vi "Test-XBoxController-Virtual.vi"() -> ()   [LabVIEW 2013]
uses:
  Robot/Virtual Systems/Tracer-V/Tracer-V.lvclass
  Robot/Logical Systems/TraceMessage/Trace.lvclass
  Robot/Virtual Systems/XBoxController-V/XboxController-V.lvclass
  <vilib>/ActorFramework/Message Queue/Message Queue.lvclass/Message Queue.ctl
  <vilib>/ActorFramework/Message Enqueuer/Message Enqueuer.lvclass/Message Enqueuer.ctl
  <vilib>/ActorFramework/Message Enqueuer/Enqueue.vi
  <vilib>/ActorFramework/Message Priority Queue/Priority Enqueue.vi
  Robot/Logical Systems/XBoxController Messages/Teleop Msg/Teleop Msg.lvclass
  <vilib>/ActorFramework/Stop Msg/Stop Msg.lvclass
  <vilib>/ActorFramework/Actor/Actor.lvclass
  <vilib>/ActorFramework/Message Queue/Message Queue.lvclass
panel:
  in  "stop 2":bool
  in  "DQ milliseconds to wait":u32=20
  out "# elements in queue":i32
  in  "Operator Controller":T1 {"Right Joystick Right" scale=-1.0..1.0; "Left Joystick Right" scale=-1.0..1.0; "Right Joystick Forward" scale=-1.0..1.0; "Left Joystick Forward" scale=-1.0..1.0}
  out "Log Time Stamp":timestamp
  out "Trace TimeTick":u32
  out "Message":string
  out "SourceVI":string
  in  "Driver Controller":T1 {"Right Joystick Right" scale=-1.0..1.0; "Left Joystick Right" scale=-1.0..1.0; "Right Joystick Forward" scale=-1.0..1.0; "Left Joystick Forward" scale=-1.0..1.0}
  in  "milliseconds to wait":u32=50
  in  "stop":bool
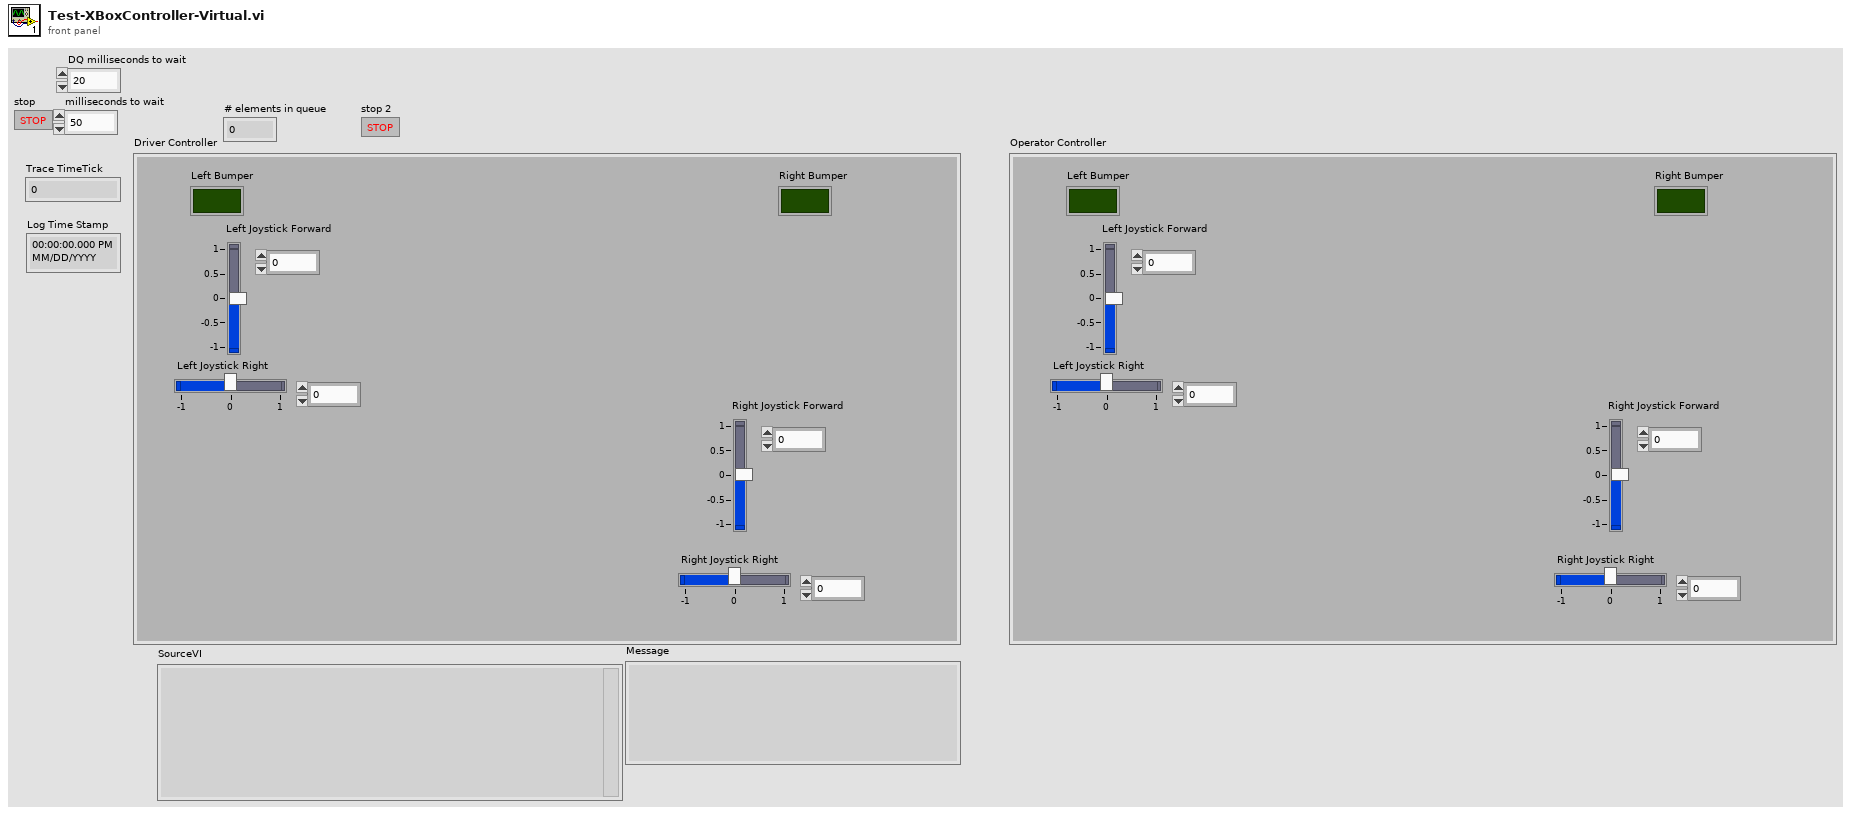
[diagram p1: front panel]
types:
  T1 = cluster{"Left Bumper":bool, "Right Bumper":bool, "Left Joystick Forward":dbl, "Left Joystick Right":dbl, "Right Joystick Forward":dbl, "Right Joystick Right":dbl}
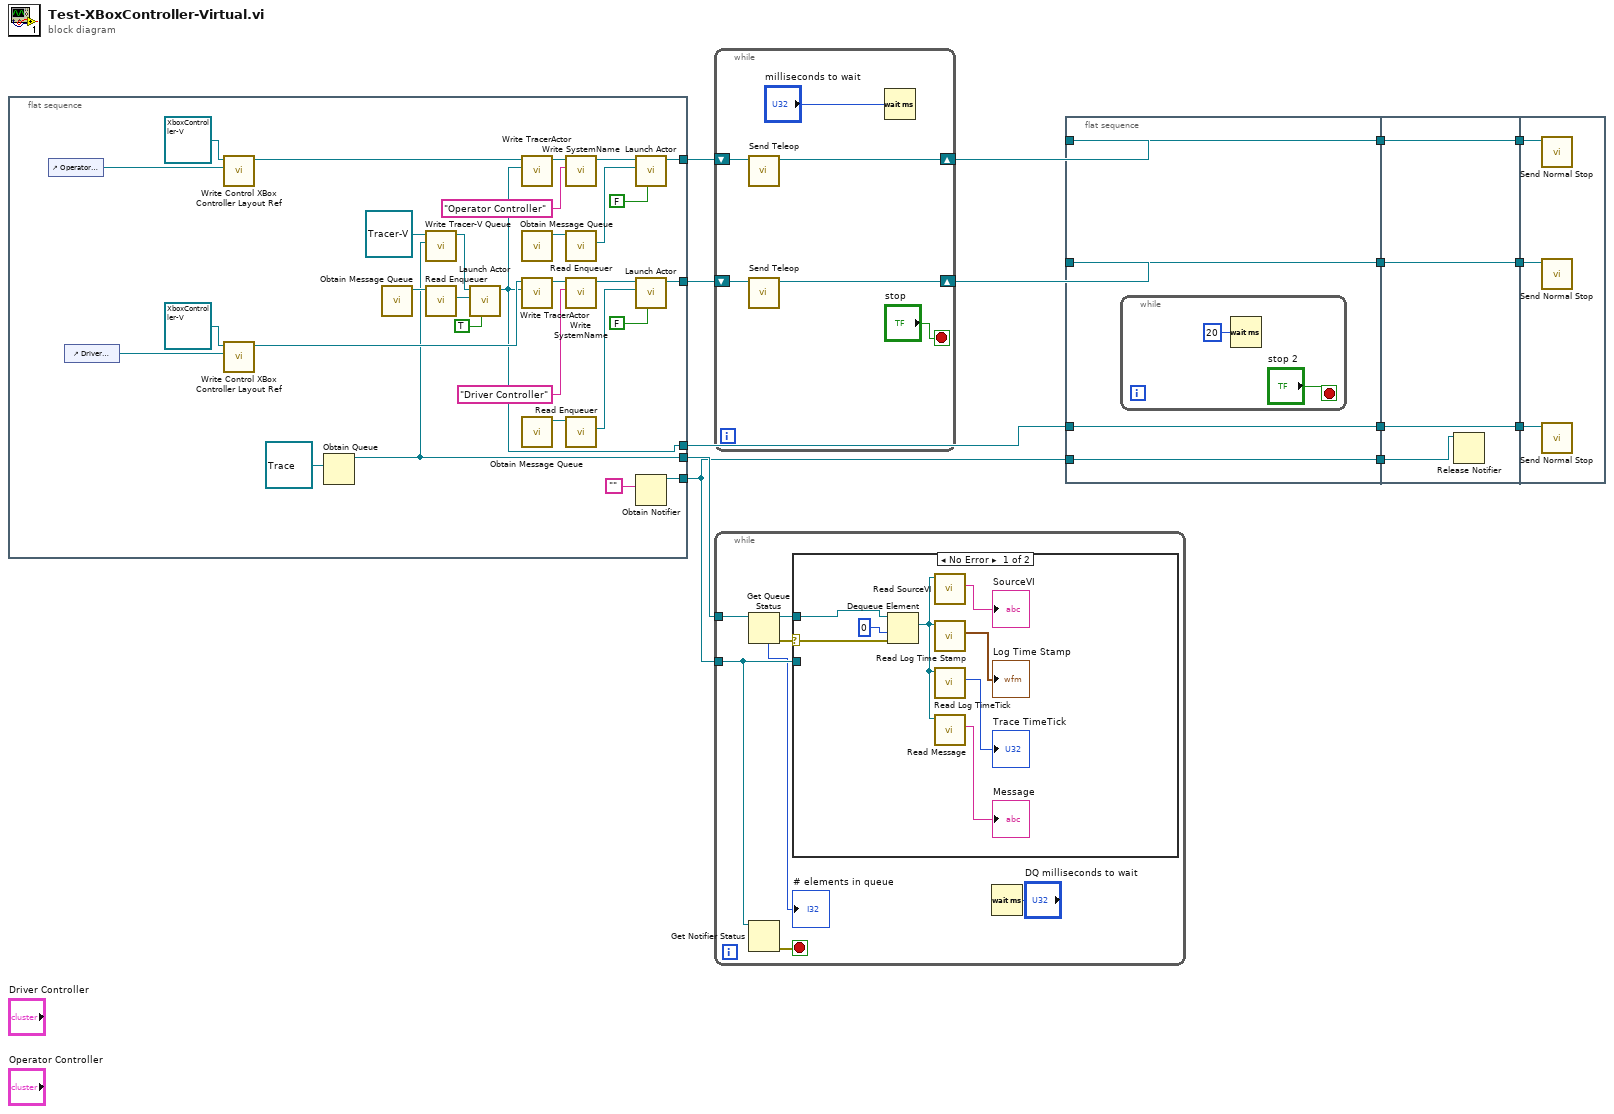
[diagram p0: block diagram]
diagram:
  n1 = flat-sequence {
    tunnel: [w42] -> w14
    tunnel: [w26] -> w12
    tunnel: [w29] -> w9
    tunnel: [w20] -> w11
    tunnel: [w17] -> w5
    frame #0 {
      n2 = control-ref of="Operator Controller"() -> (w27:refnum<vi>)
      n3 = control-ref of="Driver Controller"() -> (w39:refnum<vi>)
      n4 = call-dynamic "Write Control XBox Controller Layout Ref.vi"("XBox Controller Layout Ref"=w27, "XboxController-V in"=refnum<class "XboxController-V.lvclass"> refnum ("XboxController-V.lvclass")) -> ("XboxController-V out"=w25:refnum<class "XboxController-V.lvclass">)  [unwired: 8 in, 1 out]
      n5 = call-dynamic "Write Control XBox Controller Layout Ref.vi"("XBox Controller Layout Ref"=w39, "XboxController-V in"=refnum<class "XboxController-V.lvclass"> refnum ("XboxController-V.lvclass")) -> ("XboxController-V out"=w33:refnum<class "XboxController-V.lvclass">)  [unwired: 8 in, 1 out]
      n6 = Obtain Queue(element data type=refnum<class "Trace.lvclass"> refnum ("Trace.lvclass")) -> (queue out=w29:refnum<queue>)  [unwired: 4 in, 2 out]
      n7 = call <vilib>:"Obtain Message Queue.vi"() -> ("Message Queue"=w35:refnum<class "Message Queue.lvclass">)  [unwired: 10 in, 1 out]
      n8 = call-dynamic "Write Tracer-V Queue.vi"("TraceMessage Queue"=w29, "Tracer-V in"=refnum<class "Tracer-V.lvclass"> refnum ("Tracer-V.lvclass")) -> ("Tracer-V out"=w30:refnum<class "Tracer-V.lvclass">)  [unwired: 8 in, 1 out]
      n9 = call <vilib>:"Read Enqueuer.vi"("Message Queue"=w35) -> ("Message Enqueuer"=w34:refnum<class "Message Enqueuer.lvclass">)  [unwired: 10 in]
      n10 = call <vilib>:"Launch Actor.vi"("Open Actor Core front panel? (F)"=TRUE, "Actor-to-Caller Enqueuer"=w34, "Actor"=w30) -> ("Caller-To-Actor Enqueuer"=w26:refnum<class "Message Enqueuer.lvclass">)  [unwired: 7 in, 1 out]
      n11 = call-dynamic "Write TracerActor.vi"("Tracer"=w26, "System in"=w25) -> ("System out"=w24:refnum<class "XboxController-V.lvclass">)  [unwired: 8 in, 1 out]
      n12 = call <vilib>:"Obtain Message Queue.vi"() -> ("Message Queue"=w22:refnum<class "Message Queue.lvclass">)  [unwired: 10 in, 1 out]
      n13 = call-dynamic "Write TracerActor.vi"("Tracer"=w26, "System in"=w33) -> ("System out"=w36:refnum<class "XboxController-V.lvclass">)  [unwired: 8 in, 1 out]
      n14 = call <vilib>:"Obtain Message Queue.vi"() -> ("Message Queue"=w44:refnum<class "Message Queue.lvclass">)  [unwired: 10 in, 1 out]
      n15 = call-dynamic "Write SystemName.vi"("SystemName"="Operator Controller", "System in"=w24) -> ("System out"=w23:refnum<class "XboxController-V.lvclass">)  [unwired: 8 in, 1 out]
      n16 = call <vilib>:"Read Enqueuer.vi"("Message Queue"=w22) -> ("Message Enqueuer"=w21:refnum<class "Message Enqueuer.lvclass">)  [unwired: 10 in]
      n17 = call-dynamic "Write SystemName.vi"("SystemName"="Driver Controller", "System in"=w36) -> ("System out"=w38:refnum<class "XboxController-V.lvclass">)  [unwired: 8 in, 1 out]
      n18 = call <vilib>:"Read Enqueuer.vi"("Message Queue"=w44) -> ("Message Enqueuer"=w43:refnum<class "Message Enqueuer.lvclass">)  [unwired: 10 in]
      n19 = call <vilib>:"Launch Actor.vi"("Open Actor Core front panel? (F)"=FALSE, "Actor-to-Caller Enqueuer"=w21, "Actor"=w23) -> ("Caller-To-Actor Enqueuer"=w20:refnum<class "Message Enqueuer.lvclass">)  [unwired: 7 in, 1 out]
      n20 = call <vilib>:"Launch Actor.vi"("Open Actor Core front panel? (F)"=FALSE, "Actor-to-Caller Enqueuer"=w43, "Actor"=w38) -> ("Caller-To-Actor Enqueuer"=w42:refnum<class "Message Enqueuer.lvclass">)  [unwired: 7 in, 1 out]
      n21 = Obtain Notifier(notification data type="") -> (notifier out=w17:refnum<notifier>)  [unwired: 3 in, 2 out]
    }
  }
  n22 = while {
    shift-right: [w47] -> w13
    shift-left: w14 -> [w48]
    shift-right: [w45] -> w10
    shift-left: w11 -> [w46]
    stop <- "stop" stop-if-true
    n23 = call "Send Teleop.vi"("Message Enqueuer"=w46) -> ("Message Enqueuer out"=w45:refnum<class "Message Enqueuer.lvclass">)  [unwired: 9 in, 1 out]
    n24 = call "Send Teleop.vi"("Message Enqueuer"=w48) -> ("Message Enqueuer out"=w47:refnum<class "Message Enqueuer.lvclass">)  [unwired: 9 in, 1 out]
    n25 = Wait (ms)(milliseconds to wait="milliseconds to wait") -> ()  [unwired: 1 out]
  }
  n26 = while {
    tunnel: w9 -> [w57]
    tunnel: w5 -> [w54]
    stop <- w53 stop-if-true
    n27 = Get Queue Status(queue=w57) -> (queue out=w56:refnum<queue>, error out=w55:errorcluster, # elements in queue=→"# elements in queue":i32)  [unwired: 2 in, 5 out]
    n28 = Get Notifier Status(notifier=w54) -> (error out=w53:errorcluster)  [unwired: 1 in, 4 out]
    n29 = case shown="No Error" w55 {
      selector: w55 -> [w59 _]
      tunnel: w56 -> [w65 _]
      tunnel: w54 -> [_ _]
      frame No Error {
        n30 = Dequeue Element(queue=w65, timeout in ms (-1)=0, error in (no error)=w59) -> (element=w60:refnum<class "Trace.lvclass">)  [unwired: 3 out]
        n31 = call-dynamic "Read SourceVI.vi"("Trace in"=w60) -> ("SourceVI"=→"SourceVI":string)  [unwired: 8 in, 2 out]
        n32 = call-dynamic "Read Log Time Stamp.vi"("Trace in"=w60) -> ("Log Time Stamp"=→"Log Time Stamp":timestamp)  [unwired: 8 in, 2 out]
        n33 = call-dynamic "Read Log TimeTick.vi"("TraceMessage in"=w60) -> ("Trace TimeTick"=→"Trace TimeTick":u32)  [unwired: 8 in, 2 out]
        n34 = call-dynamic "Read Message.vi"("TraceMessage in"=w60) -> ("Message"=→"Message":string)  [unwired: 8 in, 2 out]
      }
      frame Error {
      }
    }
    n35 = Wait (ms)(milliseconds to wait="DQ milliseconds to wait") -> ()  [unwired: 1 out]
  }
  n36 = flat-sequence {
    tunnel: w5 -> [w66]
    tunnel: w10 -> [w67]
    tunnel: w12 -> [w68]
    tunnel: w13 -> [w69]
    tunnel: [w69] -> w4
    tunnel: [w68] -> w3
    tunnel: [w67] -> w2
    tunnel: [w66] -> w1
    tunnel: [w75] -> w8
    tunnel: [w74] -> w7
    tunnel: [w73] -> w6
    tunnel: w4 -> [w75]
    tunnel: w3 -> [w74]
    tunnel: w2 -> [w73]
    tunnel: w1 -> [w72]
    tunnel: w8 -> [w78]
    tunnel: w7 -> [w77]
    tunnel: w6 -> [w76]
    frame #0 {
      n37 = while {
        stop <- "stop 2" stop-if-true
        n38 = Wait (ms)(milliseconds to wait=u32 20) -> ()  [unwired: 1 out]
      }
    }
    frame #1 {
      n39 = Release Notifier(notifier=w72) -> ()  [unwired: 2 in, 3 out]
    }
    frame #2 {
      n40 = call <vilib>:"Send Normal Stop.vi"("Message Enqueuer"=w76) -> ()  [unwired: 10 in, 1 out]
      n41 = call <vilib>:"Send Normal Stop.vi"("Message Enqueuer"=w78) -> ()  [unwired: 10 in, 1 out]
      n42 = call <vilib>:"Send Normal Stop.vi"("Message Enqueuer"=w77) -> ()  [unwired: 10 in, 1 out]
    }
  }
